vi "checkSpectroConfig.vi"(8 "Error IN":errorcluster caption="constante d'erreur", 11 "Background folder path":path=path "") -> (0 "Error OUT":errorcluster caption="constante d'erreur", 1 "spectroConfigIsOk?":bool=TRUE, 3 "spectroConfig":T6)   [LabVIEW 2020]
uses:
  defTypeConfigs/spectroConfig.ctl
  defTypeConfigs/globalCAM.ctl
  defTypeConfigs/globalSTRIPS.ctl
  defTypeConfigs/globalPARAMS.ctl
  defTypeConfigs/globalSPECTRO.ctl
  defTypeConfigs/intSPECTRO.ctl
panel:
  out "Image back Handle":u32
  out "Background path file":path
  out "BackIsOK":bool
  in  "Acquire background":bool
  out "INIT SPECTRO":T1
  in  "SPECTRO PARAMETERS":T2={"Wavelength"=500.0, "Grating number"=1, "Spectro parameters updated"=FALSE, "Init spectro"=FALSE, "Background file"="Background_file", "check"=FALSE, "resultCheckBackFile"=""}
  in  "CAM PARAMETERS":T3 {"Temperature setting (°C)" step=1.0; "Temperature (°C)" step=1.0; "Exposure time (s)" min=0.0001 max=10.0 step=0.1}
  in  "Start acquisition":bool
  in  "STRIPS PARAMETERS":T4={"Strips number"=enum."12", "Y binning"=0, "Gap (%)"=0, "Init strips"=FALSE, "Strips updated"=FALSE, "max"=400.0} {"Gap (%)" max=100 step=1; "Y binning" min=1 step=1}
  out "INIT CAM":T5
  in  "Exit app":bool
  # "Spectrometer and camera\nConfiguration"
  # "Grating\nWaveLength\nAccumulations\nSample Time\nNb Frames\nNb Strip\nGap(%)\nRépertoire d'enregistrement background\nRépertoire d'enregistrement du spectre\nRépertoire de la configuration winspec"
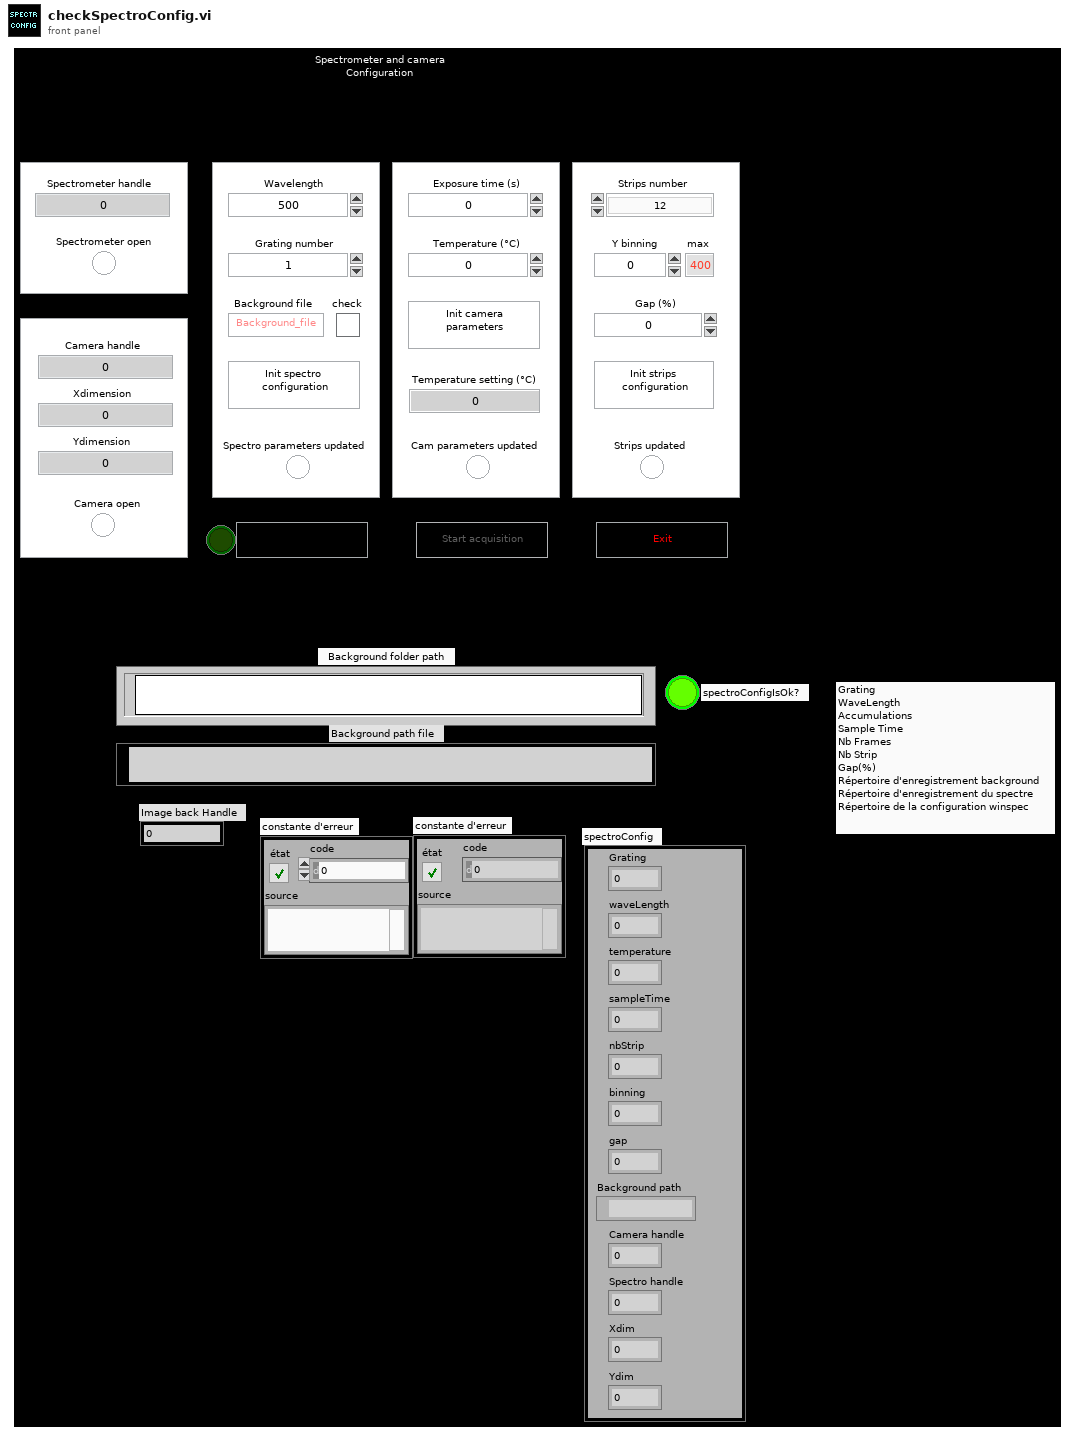
[diagram p1: front panel]
types:
  T1 = typedef "intSPECTRO.ctl" = cluster{"Spectrometer handle":i32, "Spectrometer open":bool}
  T2 = typedef "globalSPECTRO.ctl" = cluster{"Wavelength":dbl, "Grating number":u32, "Spectro parameters updated":bool, "Init spectro":bool, "Background file":string, "check":bool, "resultCheckBackFile":string}
  T3 = typedef "globalPARAMS.ctl" = cluster{"Exposure time (s)":dbl, "Init CAM":bool, "Cam parameters updated":bool, "Temperature (°C)":dbl, "Temperature setting (°C)":dbl}
  T4 = typedef "globalSTRIPS.ctl" = cluster{"Strips number":enum16{"12", "4", "2", "1"}, "Y binning":u32, "Gap (%)":u32, "Init strips":bool, "Strips updated":bool, "max":dbl}
  T5 = typedef "globalCAM.ctl" = cluster{"Ydimension":i32, "Xdimension":i32, "Camera handle":i32, "Camera open":bool}
  T6 = typedef "spectroConfig.ctl" = cluster{"Grating":i32, "waveLength":i32, "sampleTime":dbl, "nbStrip":i32, "gap":i32, "Background path":path, "temperature":dbl, "binning":i32, "Camera handle":i32, "Spectro handle":i32, "Xdim":i32, "Ydim":i32}
  T7 = enum8{"Enabled", "Disabled", "Disabled and Grayed Out"}
  T8 = cluster{"Spectrometer handle":i32, "Spectrometer open":bool}
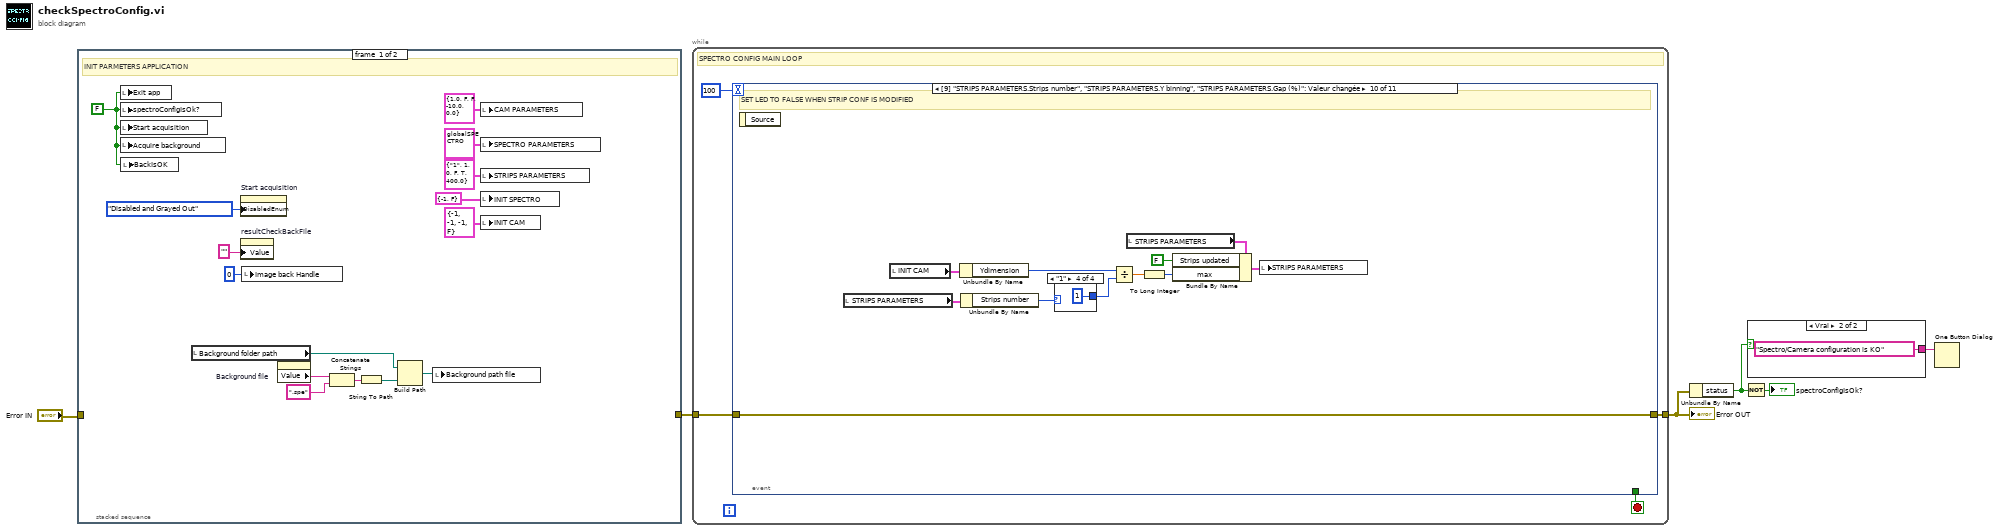
[diagram p0: block diagram]
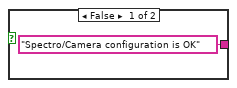
[diagram p2: hidden frame]
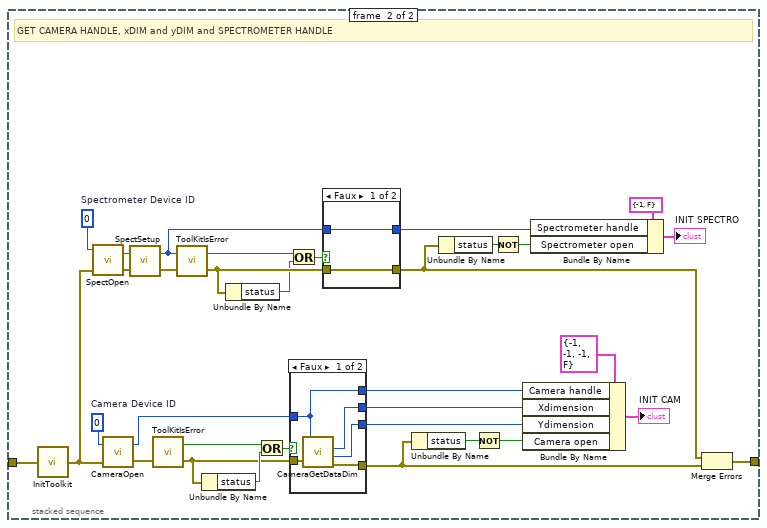
[diagram p3: hidden frame]
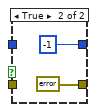
[diagram p4: hidden frame]
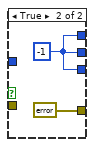
[diagram p5: hidden frame]
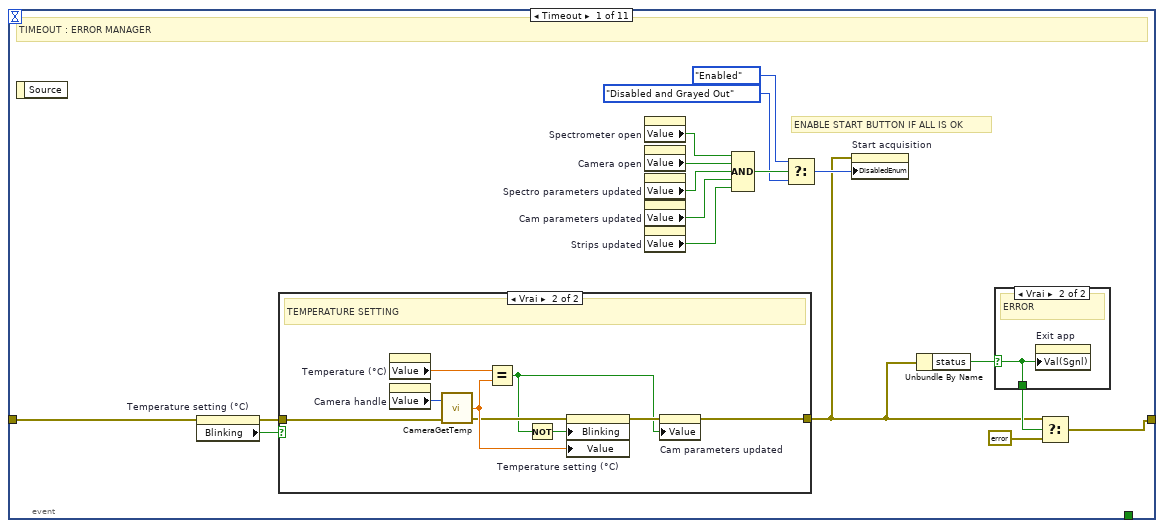
[diagram p6: hidden frame]
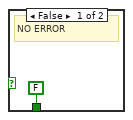
[diagram p8: hidden frame]
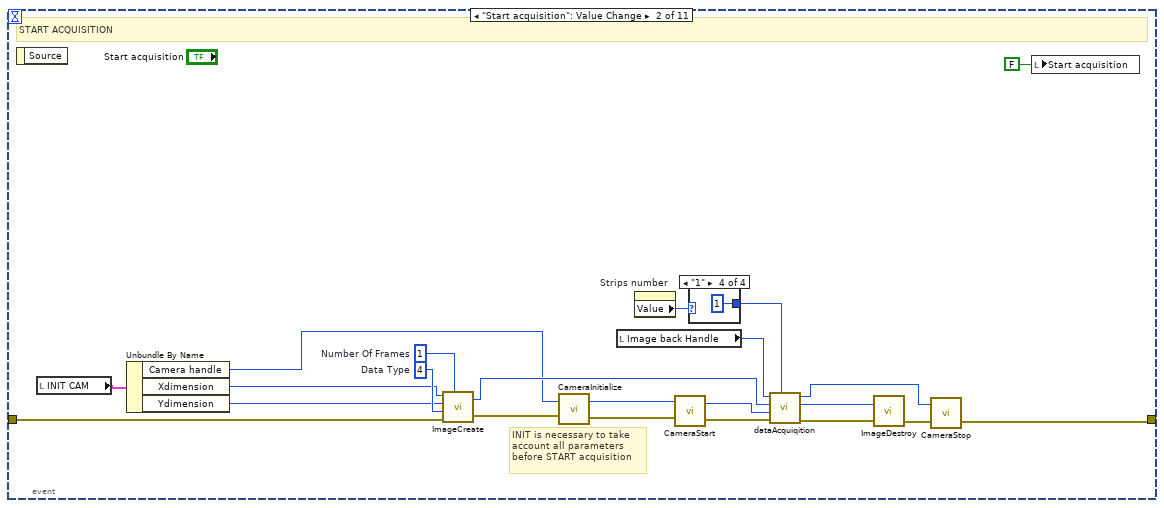
[diagram p9: hidden frame]
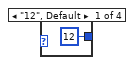
[diagram p10: hidden frame]
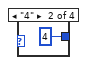
[diagram p11: hidden frame]
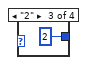
[diagram p12: hidden frame]
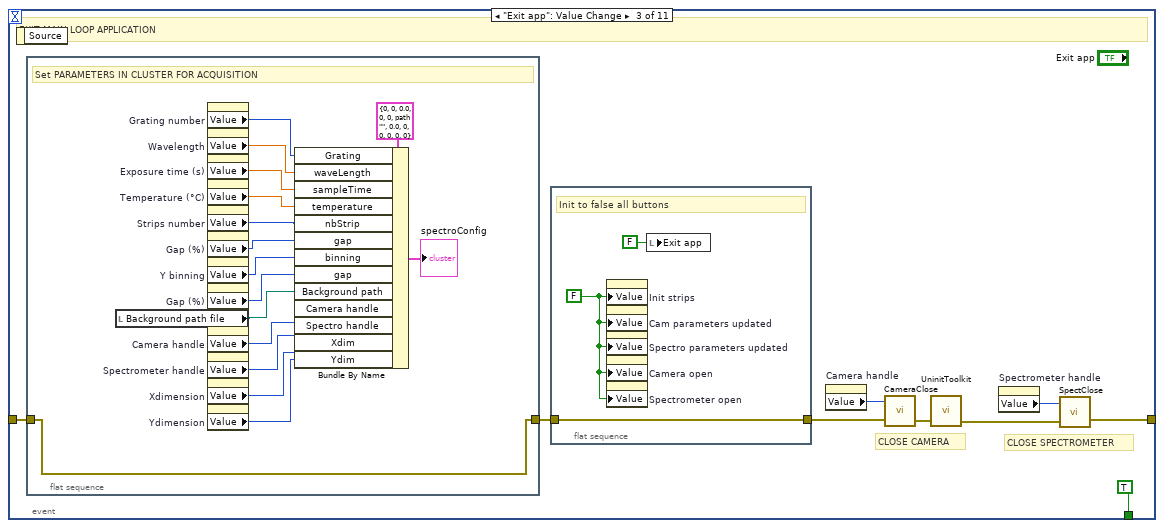
[diagram p13: hidden frame]
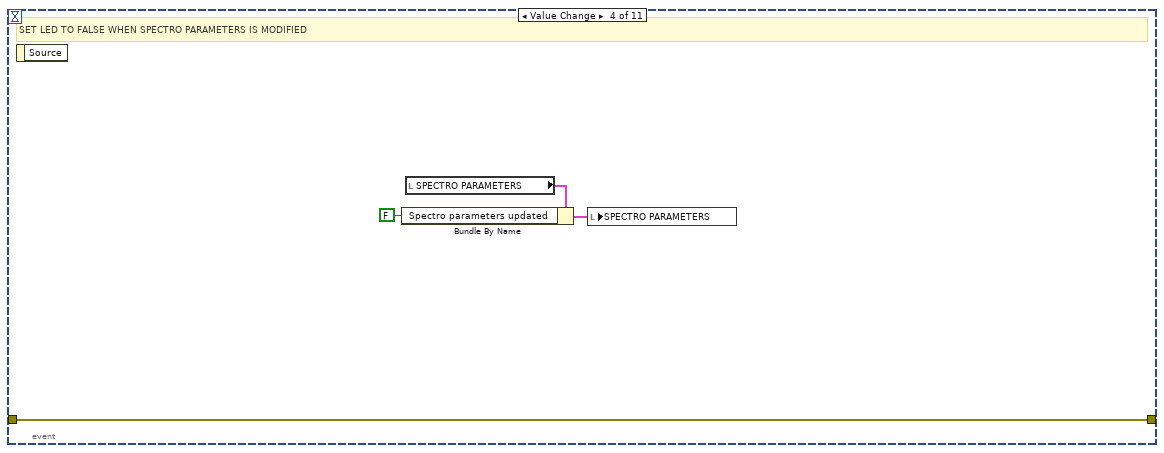
[diagram p14: hidden frame]
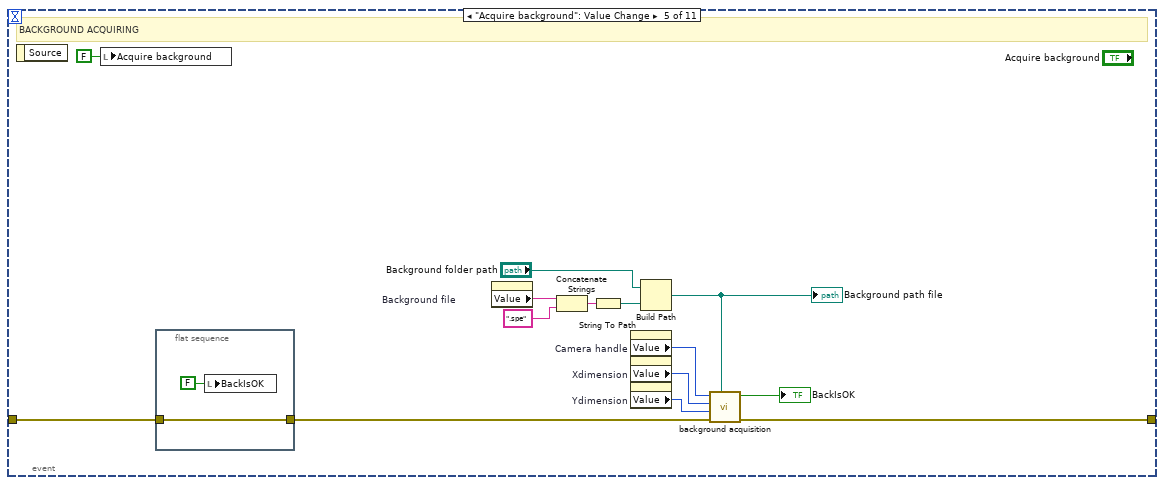
[diagram p15: hidden frame]
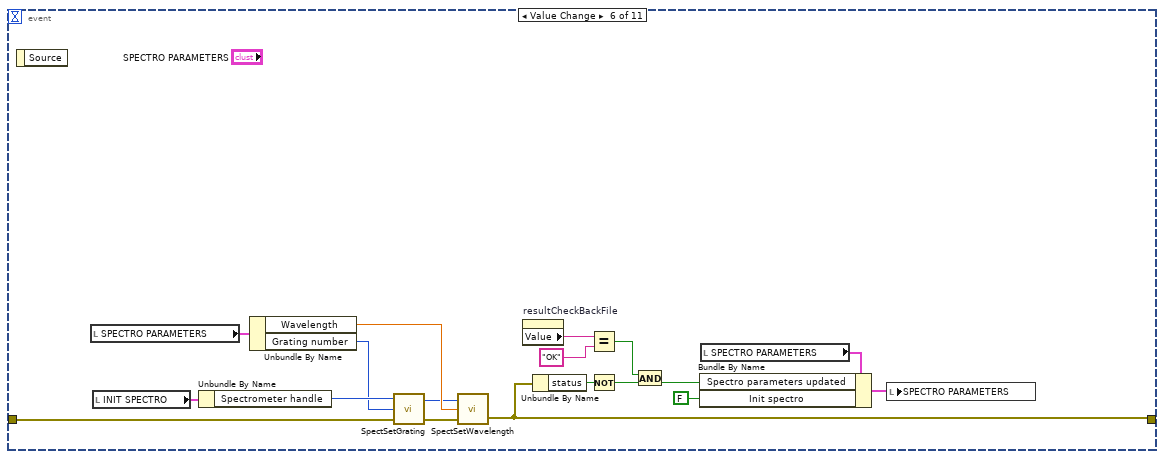
[diagram p16: hidden frame]
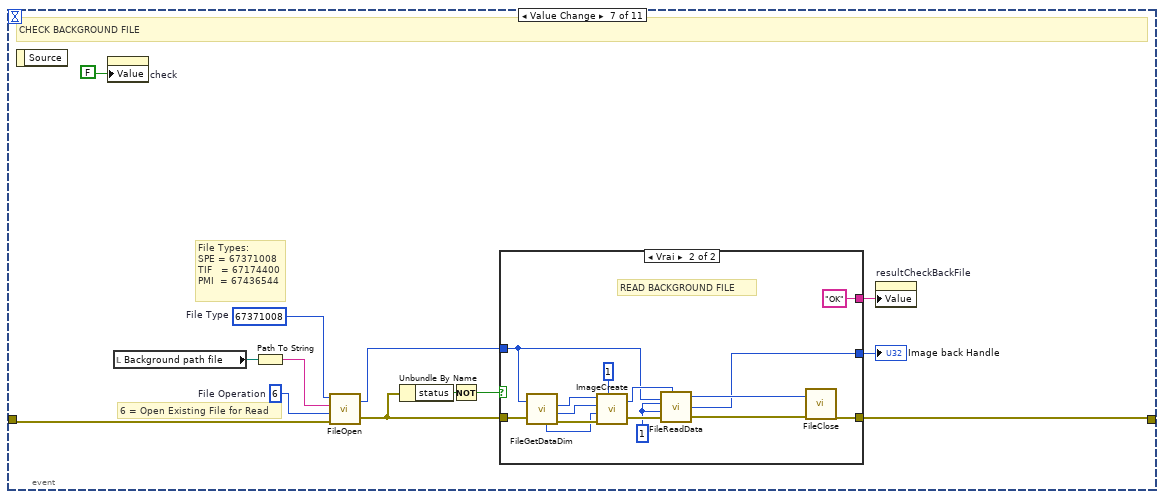
[diagram p17: hidden frame]
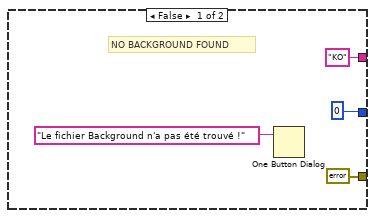
[diagram p18: hidden frame]
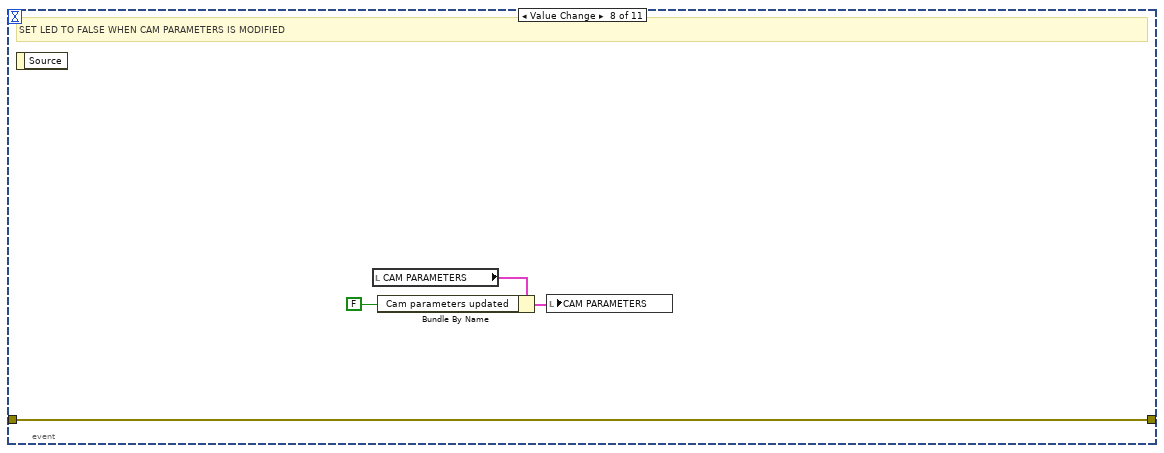
[diagram p19: hidden frame]
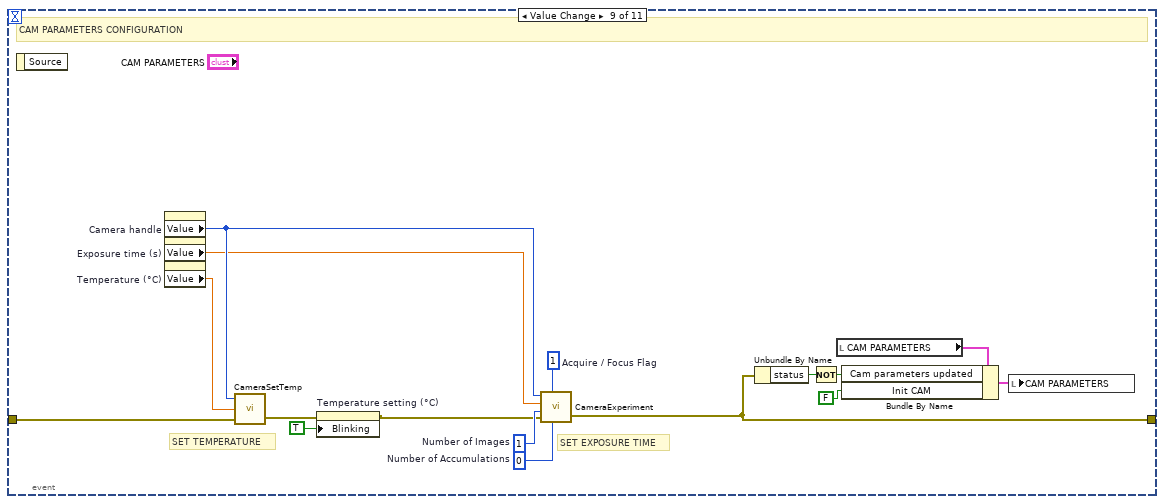
[diagram p20: hidden frame]
diagram:
  n1 = stacked-sequence {
    tunnel: "Error IN" -> [_ w53]
    tunnel: [_ w34] -> w5
    frame #0 {
      w17 = FALSE ("Exit app")
      # "INIT PARMETERS APPLICATION"
      n2 = local write "Exit app"(w17) -> ()
      n3 = local write "spectroConfigIsOk?"(w17) -> ()
      n4 = local write "Start acquisition"(w17) -> ()
      n5 = local write "Acquire background"(w17) -> ()
      n6 = local write "BackIsOK"(w17) -> ()
      n7 = local read "Background folder path"() -> (w12:path)
      n8 = property on="Start acquisition" class="Bool (strict)"("DisabledEnum"=T7."Disabled and Grayed Out" ("Désactivé")) -> ()  [unwired: 2 in, 2 out]
      n9 = property on="resultCheckBackFile" class="Ch"("Value"="" ("Valeur")) -> ()  [unwired: 2 in, 2 out]
      n10 = local write "Image back Handle"(u32 0 ("Image back Handle")) -> ()
      n11 = property on="Background file" class="Ch"() -> ("Value"=w14:string)  [unwired: 2 in, 2 out]
      n12 = Concatenate Strings(w14, ".spe" ("chaîne")) -> (w16:string)
      n13 = String To Path(string=w16) -> (path=w13:path)
      n14 = Build Path(base path=w12, name or relative path=w13) -> (appended path=w11:path)
      n15 = local write "Background path file"(w11) -> ()
      n16 = local write "CAM PARAMETERS"(T3 {"Exposure time (s)"=1.0, "Init CAM"=FALSE, "Cam parameters updated"=FALSE, "Temperature (°C)"=-10.0, "Temperature setting (°C)"=0.0} ("CAM PARAMETERS")) -> ()
      n17 = local write "SPECTRO PARAMETERS"(T2 {"Wavelength"=500.0, "Grating number"=1, "Spectro parameters updated"=FALSE, "Init spectro"=FALSE, "Background file"="Background_file", "check"=FALSE, "resultCheckBackFile"=""} ("Global SPECTRO")) -> ()
      n18 = local write "STRIPS PARAMETERS"(T4 {"Strips number"=enum."1", "Y binning"=1, "Gap (%)"=0, "Init strips"=FALSE, "Strips updated"=TRUE, "max"=400.0} ("STRIPS PARAMETERS")) -> ()
      n19 = local write "INIT SPECTRO"(T8 {"Spectrometer handle"=-1, "Spectrometer open"=FALSE} ("INIT SPECTRO")) -> ()
      n20 = local write "INIT CAM"(T5 {"Ydimension"=-1, "Xdimension"=-1, "Camera handle"=-1, "Camera open"=FALSE} ("INIT CAM")) -> ()
    }
    frame #1 {
      w40 = u32 0  # Spectrometer Device ID
      w54 = u32 0  # Camera Device ID
      # "GET CAMERA HANDLE, xDIM and yDIM and SPECTROMETER HANDLE"
      n21 = call <userlib>:"InitToolkit.vi"("error in"=w53) -> ("error out"=w39:errorcluster)
      n22 = call <userlib>:"SpectOpen.vi"("error in"=w39, "Spectrometer ID"=w40) -> ("error out"=w42:errorcluster, "Spectrometer Handle"=w41:u32)  [unwired: 1 in]
      n23 = call <userlib>:"CameraOpen.vi"("error in"=w39, "Camera Device ID"=w54) -> ("error out"=w52:errorcluster, "Camera Handle"=w50:u32)
      n24 = call <userlib>:"SpectSetup.vi"("error in"=w42, "Spectrometer Handle"=w41) -> ("error out"=w38:errorcluster, "Spectrometer Handle"=w35:u32)
      n25 = call <userlib>:"ToolKitIsError.vi"("error in"=w52) -> ("error out"=w26:errorcluster, "Error Flag"=w51:bool)  [unwired: 1 in]
      n26 = call <userlib>:"ToolKitIsError.vi"("error in"=w38, "Reserved"=w35) -> ("error out"=w23:errorcluster, "Error Flag"=w24:bool)
      n27 = Unbundle By Name(w26) -> ("status"=w27:bool)
      n28 = Unbundle By Name(w23) -> ("status"=w22:bool)
      n29 = Or(x=w51, y=w27) -> (x .or. y?=w28:bool)
      n30 = Or(x=w24, y=w22) -> (x .or. y?=w25:bool)
      n31 = case shown="Faux" w28 {
        tunnel: w50 -> [w59 _]
        tunnel: w26 -> [w63 _]
        tunnel: [w62 errorcluster {"status"=TRUE, "code"=1, "source"="Error in openning CAMERA"} ("error out")] -> w33
        tunnel: [w61 w65] -> w47
        tunnel: [w60 w65] -> w48
        tunnel: [w59 w65] -> w49
        frame False {
          n32 = call <userlib>:"CameraGetDataDim.vi"("Camera Handle"=w59, "error in"=w63) -> ("Xdim"=w60:u32, "Ydim"=w61:u32, "error out"=w62:errorcluster)  [unwired: 1 out]
        }
        frame True {
          w65 = -1 ("Xdim")
        }
      }
      n33 = case shown="Faux" w25 {
        tunnel: [w56 -1 ("Xdim")] -> w36
        tunnel: w35 -> [w56 _]
        tunnel: w23 -> [w55 _]
        tunnel: [w55 errorcluster {"status"=TRUE, "code"=2, "source"="Error in openning SPECTROMETER"} ("error out")] -> w31
        frame False {
        }
        frame True {
        }
      }
      n34 = Unbundle By Name(w33) -> ("status"=w44:bool)
      n35 = Unbundle By Name(w31) -> ("status"=w32:bool)
      n36 = Not(x=w44) -> (.not. x?=w43:bool)
      n37 = Not(x=w32) -> (.not. x?=w30:bool)
      n38 = Bundle By Name(cluster=T5 {"Ydimension"=-1, "Xdimension"=-1, "Camera handle"=-1, "Camera open"=FALSE} ("Global CAM"), "Camera handle"=w49, "Xdimension"=w48, "Ydimension"=w47, "Camera open"=w43) -> (→"INIT CAM":T5)
      n39 = Bundle By Name(cluster=T8 {"Spectrometer handle"=-1, "Spectrometer open"=FALSE} ("INIT SPECTRO"), "Spectrometer handle"=w36, "Spectrometer open"=w30) -> (→"INIT SPECTRO":T8)
      n40 = Merge Errors(w31, w33) -> (w34:errorcluster)
    }
  }
  n41 = while {
    tunnel: w5 -> [w66]
    tunnel: [w67] -> w3
    stop <- w68 stop-if-true
    # "SPECTRO CONFIG MAIN LOOP"
    n42 = event shown="[9] \"STRIPS PARAMETERS.Strips number\", \"STRIPS PARAMETERS.Y binning\", \"STRIPS PARAMETERS.Gap (%)\": Valeur changée" {
      selector: _ -> [_ _ _ _ _ _ _ _ _ _ _]
      dyn-events: _ -> [_ _ _ _ _ _ _ _ _ _ _]
      timeout: 100 -> [_ _ _ _ _ _ _ _ _ _ _]
      tunnel: [_ _ TRUE _ _ _ _ _ _ _ _] -> w68
      tunnel: w66 -> [w82 w104 w126 w153 w158 w182 w195 w223 w234 w253 w265]
      tunnel: [w85 w103 w130 w153 w169 w178 w194 w223 w237 w253 w263] -> w67
      event Timeout {
        # "ENABLE START BUTTON IF ALL IS OK"
        # "TIMEOUT : ERROR MANAGER"
        n43 = event-data() -> ()  [unwired: 1 in, 1 out]
        n44 = property on="Temperature setting (°C)" class="NumNb (strict)"(error in=w82) -> (error out=w80:errorcluster, "Blinking"=w81:bool)  [unwired: 1 in, 1 out]
        n45 = case shown="Vrai" w81 {
          tunnel: w80 -> [w87 w94]
          tunnel: [w87 w90] -> w70
          frame False {
            # "NOTHING TO DO"
          }
          frame True {
            # "TEMPERATURE SETTING"
            n46 = property on="Temperature (°C)" class="NumNb (strict)"() -> ("Value"=w95:dbl)  [unwired: 2 in, 2 out]
            n47 = property on="Camera handle" class="NumNb (strict)"() -> ("Value"=w96:i32)  [unwired: 2 in, 2 out]
            n48 = call <userlib>:"CameraGetTemp.vi"("Camera Handle"=w96, "error in (no error)"=w94) -> ("Temperature"=w93:dbl, "error out"=w92:errorcluster)  [unwired: 1 out]
            n49 = Equal?(x=w95, y=w93) -> (x = y?=w88:bool)
            n50 = Not(x=w88) -> (.not. x?=w89:bool)
            n51 = property on="Temperature setting (°C)" class="NumNb (strict)"(error in=w92, "Blinking"=w89, "Value"=w93) -> (error out=w91:errorcluster)  [unwired: 1 in, 1 out]
            n52 = property on="Cam parameters updated" class="Bool (strict)"(error in=w91, "Value"=w88) -> (error out=w90:errorcluster)  [unwired: 1 in, 1 out]
          }
        }
        n53 = property on="Spectrometer open" class="Bool (strict)"() -> ("Value"=w79:bool)  [unwired: 2 in, 2 out]
        n54 = property on="Camera open" class="Bool (strict)"() -> ("Value"=w78:bool)  [unwired: 2 in, 2 out]
        n55 = property on="Spectro parameters updated" class="Bool (strict)"() -> ("Value"=w77:bool)  [unwired: 2 in, 2 out]
        n56 = property on="Cam parameters updated" class="Bool (strict)"() -> ("Value"=w76:bool)  [unwired: 2 in, 2 out]
        n57 = property on="Strips updated" class="Bool (strict)"() -> ("Value"=w75:bool)  [unwired: 2 in, 2 out]
        n58 = Compound Arithmetic op=AND ("Opérateur arithmétique")(w79, w78, w77, w76, w75) -> (w74:bool)
        n59 = Select(t=T7."Enabled" ("Désactivé"), s=w74, f=T7."Disabled and Grayed Out" ("Désactivé")) -> (s? t:f=w73:T7)
        n60 = property on="Start acquisition" class="Bool (strict)"(error in=w70, "DisabledEnum"=w73) -> ()  [unwired: 1 in, 2 out]
        n61 = Unbundle By Name(w70) -> ("status"=w84:bool)
        n62 = case shown="Vrai" w84 {
          selector: w84 -> [_ w98]
          tunnel: [FALSE w98] -> w83
          frame False {
            # "NO ERROR"
          }
          frame True {
            # "ERROR"
            n63 = property on="Exit app" class="Bool (strict)"("Val(Sgnl)"=w98) -> ()  [unwired: 2 in, 2 out]
          }
        }
        n64 = Select(t=w70, s=w83, f=errorcluster {"status"=FALSE, "code"=0, "source"=""} ("constante d'erreur")) -> (s? t:f=w85:errorcluster)
      }
      event "Start acquisition": Value Change {
        w119 = u32 4  # Data Type
        w118 = u32 1  # Number Of Frames
        # "INIT is necessary to take \naccount all parameters\nbefore START acquisition"
        # "START ACQUISITION"
        n65 = event-data() -> ()  [unwired: 1 in, 1 out]
        n66 = local read "INIT CAM"() -> (w117:T5)
        n67 = Unbundle By Name(w117) -> ("Camera handle"=w102:i32, "Xdimension"=w116:i32, "Ydimension"=w115:i32)
        n68 = call <userlib>:"ImageCreate.vi"("X dimension"=w116, "Y dimension"=w115, "Data Type"=w119, "error in"=w104, "Number Of Frames"=w118) -> ("Image Handle"=w106:u32, "error out"=w105:errorcluster)
        n69 = call <userlib>:"CameraInitialize.vi"("error in"=w105, "Camera Handle"=w102) -> ("error out"=w111:errorcluster, "Camera Handle"=w110:u32)
        n70 = local read "Image back Handle"() -> (w101:u32)
        n71 = property on="Strips number" class="Énum (strict)"() -> ("Value"=w100:enum16{"12", "4", "2", "1"})  [unwired: 2 in, 2 out]
        n72 = call <userlib>:"CameraStart.vi"("error in"=w111, "Camera Handle"=w110) -> ("error out"=w114:errorcluster, "Camera Handle"=w113:u32)
        n73 = case shown="\"1\"" w100 {
          tunnel: [12 4 2 1] -> w99
          frame "12", Default {
          }
          frame "4" {
          }
          frame "2" {
          }
          frame "1" {
          }
        }
        n74 = call "dataAcquiqition.vi"("Background image handle"=w101, "Image Handle"=w106, "Camera Handle"=w113, "Error IN"=w114, "Strip number"=w99) -> ("Camera handle"=w108:i32, "Image Handle"=w107:u32, "Error OUT"=w109:errorcluster)  [unwired: 3 in]
        n75 = call <userlib>:"ImageDestroy.vi"("error in"=w109, "Data handle"=w107) -> ("error out"=w112:errorcluster)
        n76 = call <userlib>:"CameraStop.vi"("error in"=w112, "Camera Handle"=w108) -> ("error out"=w103:errorcluster)  [unwired: 1 out]
        n77 = local write "Start acquisition"(FALSE ("Start acquisition")) -> ()
      }
      event "Exit app": Value Change {
        # "CLOSE SPECTROMETER"
        # "CLOSE CAMERA"
        # "EXIT MAIN LOOP APPLICATION"
        n78 = event-data() -> ()  [unwired: 1 in, 1 out]
        n79 = flat-sequence {
          tunnel: [w140] -> w125
          tunnel: w126 -> [w140]
          frame #0 {
            # "Set PARAMETERS IN CLUSTER FOR ACQUISITION"
            n80 = local read "Background path file"() -> (w134:path)
            n81 = property on="Grating number" class="NumNb (strict)"() -> ("Value"=w147:u32)  [unwired: 2 in, 2 out]
            n82 = property on="Wavelength" class="NumNb (strict)"() -> ("Value"=w146:dbl)  [unwired: 2 in, 2 out]
            n83 = property on="Exposure time (s)" class="NumNb (strict)"() -> ("Value"=w145:dbl)  [unwired: 2 in, 2 out]
            n84 = property on="Temperature (°C)" class="NumNb (strict)"() -> ("Value"=w135:dbl)  [unwired: 2 in, 2 out]
            n85 = property on="Strips number" class="Énum (strict)"() -> ("Value"=w144:enum16{"12", "4", "2", "1"})  [unwired: 2 in, 2 out]
            n86 = property on="Gap (%)" class="NumNb (strict)"() -> ("Value"=w143:u32)  [unwired: 2 in, 2 out]
            n87 = property on="Y binning" class="NumNb (strict)"() -> ("Value"=w142:u32)  [unwired: 2 in, 2 out]
            n88 = property on="Gap (%)" class="NumNb (strict)"() -> ("Value"=w141:u32)  [unwired: 2 in, 2 out]
            n89 = property on="Camera handle" class="NumNb (strict)"() -> ("Value"=w138:i32)  [unwired: 2 in, 2 out]
            n90 = property on="Spectrometer handle" class="NumNb (strict)"() -> ("Value"=w139:i32)  [unwired: 2 in, 2 out]
            n91 = property on="Xdimension" class="NumNb (strict)"() -> ("Value"=w137:i32)  [unwired: 2 in, 2 out]
            n92 = property on="Ydimension" class="NumNb (strict)"() -> ("Value"=w136:i32)  [unwired: 2 in, 2 out]
            n93 = Bundle By Name(cluster=T6 {"Grating"=0, "waveLength"=0, "sampleTime"=0.0, "nbStrip"=0, "gap"=0, "Background path"=path "", "temperature"=0.0, "binning"=0, "Camera handle"=0, "Spectro handle"=0, "Xdim"=0, "Ydim"=0} ("spectroConfig"), "Grating"=w147, "waveLength"=w146, "sampleTime"=w145, "temperature"=w135, "nbStrip"=w144, "gap"=w143, "binning"=w142, "gap"=w141, "Background path"=w134, "Camera handle"=w138, "Spectro handle"=w139, "Xdim"=w137, "Ydim"=w136) -> (→"spectroConfig":T6)
          }
        }
        n94 = flat-sequence {
          tunnel: w125 -> [w151]
          tunnel: [w151] -> w127
          frame #0 {
            w152 = FALSE ("Valeur")
            # "Init to false all buttons"
            n95 = property on="Init strips" class="Bool (strict)"("Value"=w152) -> ()  [unwired: 2 in, 2 out]
            n96 = property on="Cam parameters updated" class="Bool (strict)"("Value"=w152) -> ()  [unwired: 2 in, 2 out]
            n97 = property on="Spectro parameters updated" class="Bool (strict)"("Value"=w152) -> ()  [unwired: 2 in, 2 out]
            n98 = property on="Camera open" class="Bool (strict)"("Value"=w152) -> ()  [unwired: 2 in, 2 out]
            n99 = property on="Spectrometer open" class="Bool (strict)"("Value"=w152) -> ()  [unwired: 2 in, 2 out]
            n100 = local write "Exit app"(FALSE ("Exit app")) -> ()
          }
        }
        n101 = property on="Camera handle" class="NumNb (strict)"() -> ("Value"=w129:i32)  [unwired: 2 in, 2 out]
        n102 = call <userlib>:"CameraClose.vi"("error in"=w127, "Camera Handle"=w129) -> ("error out"=w132:errorcluster)
        n103 = call <userlib>:"UninitToolkit.vi"("error in"=w132) -> ("error out"=w131:errorcluster)
        n104 = property on="Spectrometer handle" class="NumNb (strict)"() -> ("Value"=w128:i32)  [unwired: 2 in, 2 out]
        n105 = call <userlib>:"SpectClose.vi"("error in"=w131, "Spectrometer Handle"=w128) -> ("error out"=w130:errorcluster)
      }
      event Value Change {
        # "SET LED TO FALSE WHEN SPECTRO PARAMETERS IS MODIFIED"
        n106 = event-data() -> ()  [unwired: 1 in, 1 out]
        n107 = local read "SPECTRO PARAMETERS"() -> (w156:T2)
        n108 = Bundle By Name(cluster=w156, "Spectro parameters updated"=FALSE ("stripCongIsOK?")) -> (w155:T2)
        n109 = local write "SPECTRO PARAMETERS"(w155) -> ()
      }
      event "Acquire background": Value Change {
        # "BACKGROUND ACQUIRING"
        n110 = event-data() -> ()  [unwired: 1 in, 1 out]
        n111 = local write "Acquire background"(FALSE ("Acquire background")) -> ()
        n112 = flat-sequence {
          tunnel: w158 -> [w171]
          tunnel: [w171] -> w157
          frame #0 {
            n113 = local write "BackIsOK"(FALSE ("BackIsOK")) -> ()
          }
        }
        n114 = property on="Background file" class="Ch"() -> ("Value"=w161:string)  [unwired: 2 in, 2 out]
        n115 = Concatenate Strings(w161, ".spe" ("chaîne")) -> (w159:string)
        n116 = String To Path(string=w159) -> (path=w167:path)
        n117 = property on="Camera handle" class="NumNb (strict)"() -> ("Value"=w166:i32)  [unwired: 2 in, 2 out]
        n118 = property on="Xdimension" class="NumNb (strict)"() -> ("Value"=w165:i32)  [unwired: 2 in, 2 out]
        n119 = property on="Ydimension" class="NumNb (strict)"() -> ("Value"=w164:i32)  [unwired: 2 in, 2 out]
        n120 = Build Path(base path="Background folder path", name or relative path=w167) -> (appended path=w163:path)
        "Background path file" <- w163
        n121 = call "background acquisition.vi"("File path"=w163, "Error IN"=w157, "Ydim"=w164, "Xdim"=w165, "Camera Handle"=w166) -> ("Error OUT"=w169:errorcluster, "BackIsOK"=→"BackIsOK":bool)  [unwired: 5 in]
      }
      event Value Change {
        n122 = event-data() -> ()  [unwired: 1 in, 1 out]
        n123 = local read "SPECTRO PARAMETERS"() -> (w181:T2)
        n124 = local read "INIT SPECTRO"() -> (w185:T1)
        n125 = Unbundle By Name(w185) -> ("Spectrometer handle"=w184:i32)
        n126 = Unbundle By Name(w181) -> ("Wavelength"=w179:dbl, "Grating number"=w180:u32)
        n127 = call <userlib>:"SpectSetGrating.vi"("error in"=w182, "Grating Number"=w180, "Sepctrometer Handle"=w184) -> ("error out"=w183:errorcluster, "Spectrometer Handle"=w177:u32)
        n128 = call <userlib>:"SpectSetWavelength.vi"("error in"=w183, "Wavelength"=w179, "Spectrometer Handle"=w177) -> ("error out"=w178:errorcluster)  [unwired: 1 out]
        n129 = property on="resultCheckBackFile" class="Ch"() -> ("Value"=w175:string)  [unwired: 2 in, 2 out]
        n130 = Unbundle By Name(w178) -> ("status"=w188:bool)
        n131 = Equal?(x=w175, y="OK") -> (x = y?=w173:bool)
        n132 = Not(x=w188) -> (.not. x?=w187:bool)
        n133 = And(x=w173, y=w187) -> (x .and. y?=w176:bool)
        n134 = local read "SPECTRO PARAMETERS"() -> (w190:T2)
        n135 = Bundle By Name(cluster=w190, "Spectro parameters updated"=w176, "Init spectro"=FALSE ("initParams")) -> (w189:T2)
        n136 = local write "SPECTRO PARAMETERS"(w189) -> ()
      }
      event Value Change {
        w196 = 67371008  # File Type
        w197 = u32 6  # File Operation
        # "6 = Open Existing File for Read"
        # "File Types:\nSPE = 67371008\nTIF   = 67174400\nPMI  = 67436544"
        # "CHECK BACKGROUND FILE"
        n137 = event-data() -> ()  [unwired: 1 in, 1 out]
        n138 = property on="check" class="Bool (strict)"("Value"=FALSE ("Valeur")) -> ()  [unwired: 2 in, 2 out]
        n139 = local read "Background path file"() -> (w202:path)
        n140 = Path To String(path=w202) -> (string=w201:string)
        n141 = call <userlib>:"FileOpen.vi"("error in"=w195, "File Operations"=w197, "FileName"=w201, "File Type"=w196) -> ("error out"=w200:errorcluster, "File Handle"=w203:u32)
        n142 = Unbundle By Name(w200) -> ("status"=w199:bool)
        n143 = Not(x=w199) -> (.not. x?=w198:bool)
        n144 = case shown="Vrai" w198 {
          tunnel: [u32 0 ("Image Handle") w212] -> w193
          tunnel: w203 -> [_ w210]
          tunnel: [errorcluster {"status"=FALSE, "code"=0, "source"=""} ("error out") w211] -> w194
          tunnel: w200 -> [_ w209]
          tunnel: ["KO" "OK"] -> w191
          frame False {
            # "NO BACKGROUND FOUND"
            n145 = One Button Dialog(message="Le fichier Background n'a pas été trouvé !") -> ()  [unwired: 1 in, 1 out]
          }
          frame True {
            w215 = 1 ("End Frame")
            # "READ BACKGROUND FILE"
            n146 = call <userlib>:"FileGetDataDim.vi"("File Handle"=w210, "error in"=w209) -> ("Data Type"=w221:u32, "X dim"=w217:u32, "Y dim"=w218:u32, "error out"=w222:errorcluster)  [unwired: 2 out]
            n147 = call <userlib>:"ImageCreate.vi"("X dimension"=w217, "Y dimension"=w218, "Data Type"=w221, "error in"=w222, "Number Of Frames"=1) -> ("Image Handle"=w216:u32, "error out"=w219:errorcluster)
            n148 = call <userlib>:"FileReadData.vi"("File Handle"=w210, "Start Frame"=w215, "End Frame"=w215, "error in"=w219, "Image Handle"=w216) -> ("File Handle"=w213:u32, "Image Handle"=w212:u32, "error out"=w214:errorcluster)
            n149 = call <userlib>:"FileClose.vi"("error in"=w214, "File Handle"=w213) -> ("error out"=w211:errorcluster)
          }
        }
        "Image back Handle" <- w193
        n150 = property on="resultCheckBackFile" class="Ch"("Value"=w191) -> ()  [unwired: 2 in, 2 out]
      }
      event Value Change {
        # "SET LED TO FALSE WHEN CAM PARAMETERS IS MODIFIED"
        n151 = event-data() -> ()  [unwired: 1 in, 1 out]
        n152 = local read "CAM PARAMETERS"() -> (w226:T3)
        n153 = Bundle By Name(cluster=w226, "Cam parameters updated"=FALSE ("stripCongIsOK?")) -> (w225:T3)
        n154 = local write "CAM PARAMETERS"(w225) -> ()
      }
      event Value Change {
        w238 = u32 0  # Number of Accumulations
        w239 = u32 1  # Number of Images
        w240 = u32 1  # Acquire / Focus Flag
        # "SET EXPOSURE TIME"
        # "SET TEMPERATURE"
        # "CAM PARAMETERS CONFIGURATION"
        n155 = event-data() -> ()  [unwired: 1 in, 1 out]
        n156 = property on="Camera handle" class="NumNb (strict)"() -> ("Value"=w233:i32)  [unwired: 2 in, 2 out]
        n157 = property on="Exposure time (s)" class="NumNb (strict)"() -> ("Value"=w232:dbl)  [unwired: 2 in, 2 out]
        n158 = property on="Temperature (°C)" class="NumNb (strict)"() -> ("Value"=w231:dbl)  [unwired: 2 in, 2 out]
        n159 = call <userlib>:"CameraSetTemp.vi"("error in (no error)"=w234, "Temperature"=w231, "Camera Handle"=w233) -> ("error out"=w229:errorcluster)  [unwired: 1 out]
        n160 = property on="Temperature setting (°C)" class="NumNb (strict)"(error in=w229, "Blinking"=TRUE ("Clignotant")) -> (error out=w228:errorcluster)  [unwired: 1 in, 1 out]
        n161 = call <userlib>:"CameraExperiment.vi"("Number of Accumulations"=w238, "Acquire / Focus Flag"=w240, "error in"=w228, "Number of Images"=w239, "Exposure (sec)"=w232, "Camera Handle"=w233) -> ("error out"=w237:errorcluster)  [unwired: 1 out]
        n162 = Unbundle By Name(w237) -> ("status"=w236:bool)
        n163 = Not(x=w236) -> (.not. x?=w235:bool)
        n164 = local read "CAM PARAMETERS"() -> (w242:T3)
        n165 = Bundle By Name(cluster=w242, "Cam parameters updated"=w235, "Init CAM"=FALSE ("initParams")) -> (w241:T3)
        n166 = local write "CAM PARAMETERS"(w241) -> ()
      }
      event Value Change {
        # "SET LED TO FALSE WHEN STRIP CONF IS MODIFIED"
        n167 = event-data() -> ()  [unwired: 1 in, 1 out]
        n168 = local read "STRIPS PARAMETERS"() -> (w248:T4)
        n169 = local read "INIT CAM"() -> (w249:T5)
        n170 = Unbundle By Name(w249) -> ("Ydimension"=w247:i32)
        n171 = Unbundle By Name(w248) -> ("Strips number"=w246:enum16{"12", "4", "2", "1"})
        n172 = case shown="\"1\"" w246 {
          tunnel: [12 4 2 1] -> w245
          frame "12", Default {
          }
          frame "4" {
          }
          frame "2" {
          }
          frame "1" {
          }
        }
        n173 = Divide(x=w247, y=w245) -> (x/y=w244:dbl)
        n174 = local read "STRIPS PARAMETERS"() -> (w252:T4)
        n175 = To Long Integer(number=w244) -> (32bit integer=w243:i32)
        n176 = Bundle By Name(cluster=w252, "Strips updated"=FALSE ("stripCongIsOK?"), "max"=w243) -> (w251:T4)
        n177 = local write "STRIPS PARAMETERS"(w251) -> ()
      }
      event Value Change {
        # "BUILD AND CONFIGURE STRIPS"
        n178 = event-data() -> ()  [unwired: 1 in, 1 out]
        n179 = local read "INIT CAM"() -> (w266:T5)
        n180 = Unbundle By Name(w266) -> ("Camera handle"=w260:i32)
        n181 = call "setupCam.vi"("Error IN"=w265, "Camera Handle"=w260) -> ("error out"=w264:errorcluster)  [unwired: 1 in]
        n182 = local read "STRIPS PARAMETERS"() -> (w258:T4)
        n183 = local read "INIT CAM"() -> (w259:T5)
        n184 = call "StripsBuilder.vi"("Error IN"=w264, "Global STRIPS"=w258, "Global CAM"=w259) -> ("Error OUT"=w263:errorcluster)  [unwired: 8 in]
        n185 = Unbundle By Name(w263) -> ("status"=w262:bool)
        n186 = local read "STRIPS PARAMETERS"() -> (w269:T4)
        n187 = Not(x=w262) -> (.not. x?=w261:bool)
        n188 = Bundle By Name(cluster=w269, "Strips updated"=w261, "Init strips"=FALSE ("updateStripConfig")) -> (w268:T4)
        n189 = local write "STRIPS PARAMETERS"(w268) -> ()
      }
    }
  }
  "Error OUT" <- w3
  n190 = Unbundle By Name(w3) -> ("status"=w1:bool)
  n191 = Not(x=w1) -> (.not. x?=→"spectroConfigIsOk?":bool)
  n192 = case shown="Vrai" w1 {
    tunnel: ["Spectro/Camera configuration is OK" ("message") "Spectro/Camera configuration is KO" ("message")] -> w2
    frame False {
    }
    frame True {
    }
  }
  n193 = One Button Dialog ("Boîte de dialogue à un bouton")(message=w2) -> ()  [unwired: 1 in, 1 out]
